vi "SetPageProperty.vi"(8 "error in":errorcluster, 9 "variant":variant, 11 "This VI":refnum<vi>) -> (0 "error out":errorcluster)   [LabVIEW 2015, in "SLSC Module Template System Explorer.lvlib"]
uses:
  SLSC Module Template System Explorer.lvlib
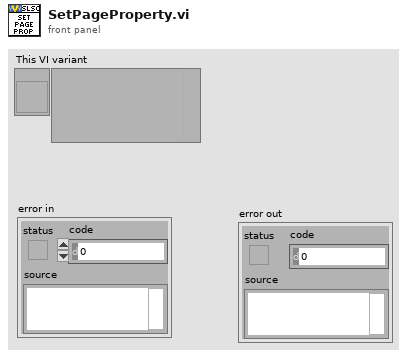
[diagram p1: front panel]
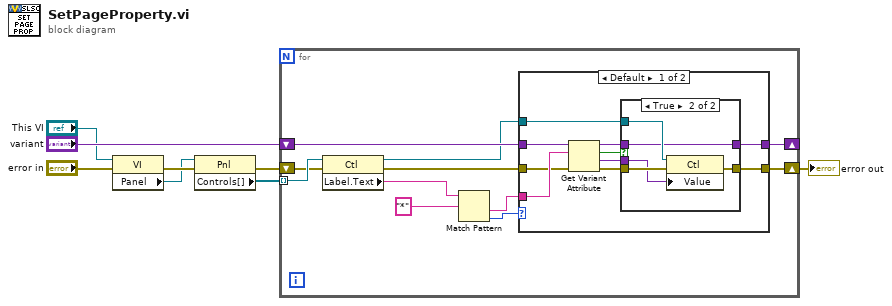
[diagram p0: block diagram]
diagram:
  n1 = property class="VI"(reference="This VI", error in="error in") -> (error out=w6:errorcluster, "Panel"=w5:refnum<vi>)  [unwired: 1 out]
  n2 = property class="Pnl"(reference=w5, error in=w6) -> (error out=w2:errorcluster, "Controls[]"=w4:refnum<vi>[])  [unwired: 1 out]
  n3 = for {
    shift-right: [w14] -> _
    shift-left: "variant" -> [w15]
    shift-right: [w16] -> w1
    shift-left: w2 -> [w17]
    tunnel: w4 -> [w18] mode=indexing
    n4 = property class="Ctl"(reference=w18, error in=w17) -> (reference out=w13:refnum<vi>, error out=w19:errorcluster, "Label.Text"=w10:string)
    n5 = Match Pattern(string=w10, regular expression="*") -> (after substring=w12:string, offset past match=w11:i32)  [unwired: 1 in, 2 out]
    n6 = case shown="Default" w11 {
      tunnel: w12 -> [w28 _]
      tunnel: w15 -> [w29 w38]
      tunnel: w19 -> [w27 w37]
      tunnel: [w21 w38] -> w14
      tunnel: [w25 w37] -> w16
      tunnel: w13 -> [w24 _]
      frame Default {
        n7 = Get Variant Attribute(Variant=w29, name=w28, error in=w27) -> (duplicate Variant=w20:variant, found=w22:bool, value=w23:variant, error out=w26:errorcluster)  [unwired: 1 in]
        n8 = case shown="True" w22 {
          tunnel: w26 -> [w30 w36]
          tunnel: [w30 w35] -> w25
          tunnel: w24 -> [_ w34]
          tunnel: w23 -> [_ w33]
          tunnel: [w31 w32] -> w21
          tunnel: w20 -> [w31 w32]
          frame False {
          }
          frame True {
            n9 = property class="Ctl"(reference=w34, error in=w36, "Value"=w33) -> (error out=w35:errorcluster)  [unwired: 1 out]
          }
        }
      }
      frame -1 {
      }
    }
  }
  "error out" <- w1
